vi "ATF-Storage-DI Cumulative Sequence Check.vi"(6 "output cluster":T1, 9 "CDT":dbl, 11 "Numeric 2":i32) -> (1 "Failure case Seq":string, 2 "Boolean":bool, 3 "String":string)   [LabVIEW 2022 SP3]
uses:
  RT Controls/ATF Storage-FGV Read write.ctl
panel:
  out "Numeric":i32
  out "number":dbl
  out "x >= y?":bool
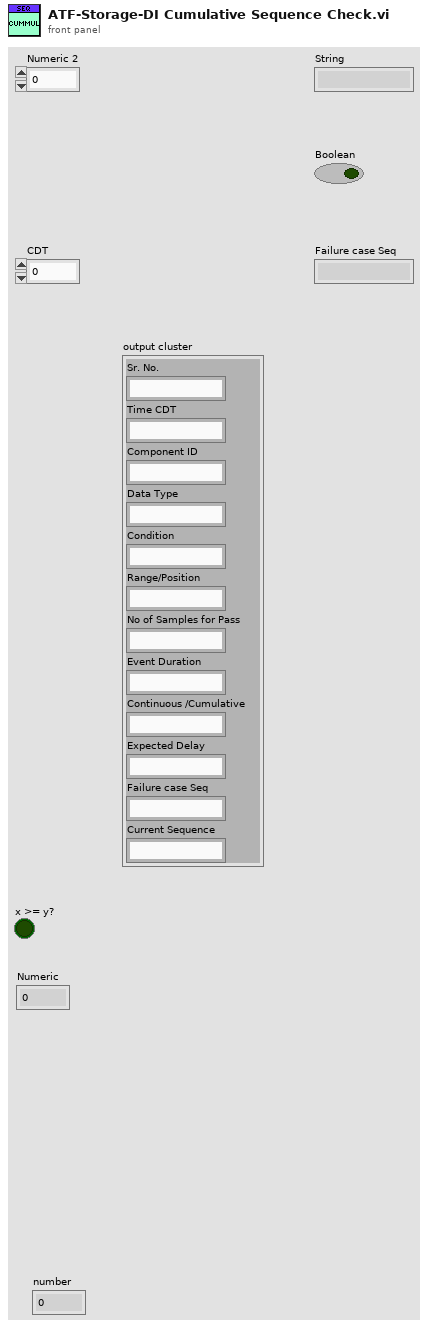
[diagram p1: front panel]
types:
  T1 = cluster{"Sr. No.":string, "Time CDT":string, "Component ID":string, "Data Type":string, "Condition":string, "Range/Position":string, "No of Samples for Pass":string, "Event Duration":string, "Continuous /Cumulative":string, "Expected Delay":string, "Failure case Seq":string, "Current Sequence":string}
  T2 = typedef "ATF Storage-FGV Read write.ctl" = enum16{"Write", "Read"}
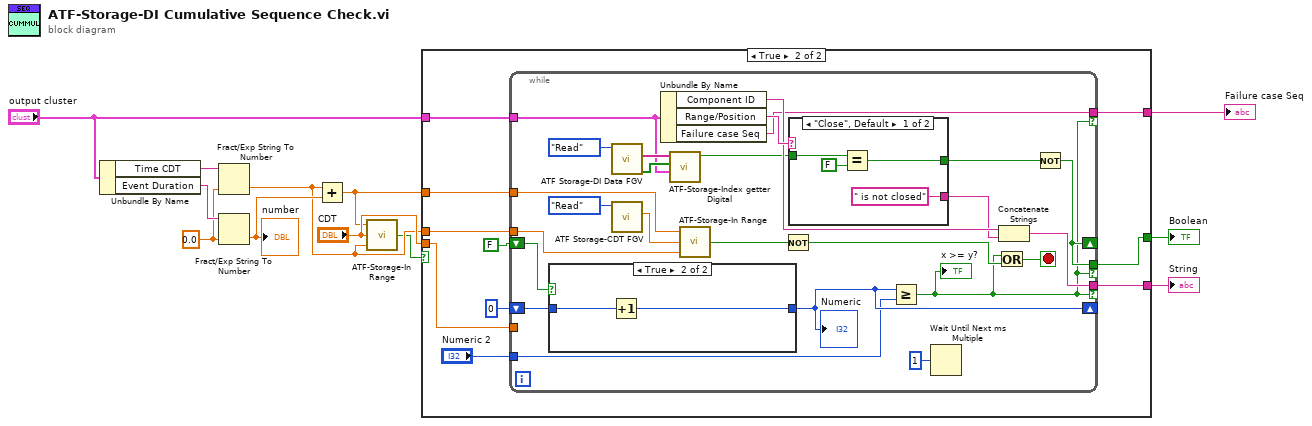
[diagram p0: block diagram]
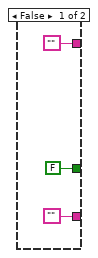
[diagram p2: hidden frame]
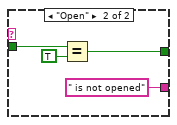
[diagram p3: hidden frame]
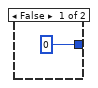
[diagram p4: hidden frame]
diagram:
  w6 = 0.0
  n1 = Unbundle By Name("output cluster") -> ("Time CDT"=w8:string, "Event Duration"=w7:string)
  n2 = Fract/Exp String To Number(string=w8, default (0 dbl)=w6) -> (number=w2:dbl)  [unwired: 2 in, 1 out]
  n3 = Fract/Exp String To Number(string=w7, default (0 dbl)=w6) -> (number=w9:dbl)  [unwired: 2 in, 1 out]
  "number" <- w9
  n4 = Add(x=w2, y=w9) -> (x+y=w3:dbl)
  n5 = call "ATF-Storage-In Range.vi"("Min"=w2, "X"="CDT", "Max"=w3) -> ("In Range"=w1:bool)  [unwired: 2 in]
  n6 = case shown="True" w1 {
    tunnel: ["" ("Empty String Constant") w25] -> w12
    tunnel: ["" ("Empty String Constant") w24] -> w11
    tunnel: [FALSE w23] -> w10
    tunnel: "output cluster" -> [_ w21]
    tunnel: "CDT" -> [_ w20]
    tunnel: w3 -> [_ w17]
    tunnel: w2 -> [_ w16]
    frame False {
    }
    frame True {
      n7 = while {
        tunnel: w21 -> [w28]
        tunnel: [w48] -> w24 if=w34
        shift-right: [w43] -> _
        shift-left: FALSE -> [w46]
        shift-right: [w45] -> _
        shift-left: 0 ("Numeric") -> [w47]
        tunnel: [w44] -> w25 if=w34
        tunnel: [w43] -> w23 if=w34
        tunnel: w20 -> [_]
        tunnel: "Numeric 2" -> [w40]
        tunnel: w17 -> [w37]
        tunnel: w16 -> [w36]
        stop <- w33 stop-if-true
        n8 = case shown="True" w46 {
          tunnel: [0 w61] -> w45
          tunnel: w47 -> [_ w60]
          frame False {
          }
          frame True {
            n9 = Increment(x=w60) -> (x+1=w61:i32)
          }
        }
        "Numeric" <- w45
        n10 = call "ATF Storage-DI Data FGV.vi"("Write/Read"=ATF_Storage-FGV_Read_write."Read") -> ("DI Y LP"=w29:bool[], "DI Signal List LP"=w30:string[])  [unwired: 8 in, 1 out]
        n11 = call "ATF Storage-CDT FGV.vi"("Write/Read"=enum16{"Write", "Read"}."Read") -> ("CDT Out"=w38:dbl)  [unwired: 9 in, 1 out]
        n12 = Unbundle By Name(w28) -> ("Component ID"=w49:string, "Range/Position"=w50:string, "Failure case Seq"=w44:string)
        n13 = call "ATF-Storage-Index getter  Digital.vi"("output cluster"=w28, "DI Y  data"=w29, "DI Channels Name"=w30) -> ("Digital data"=w27:bool)  [unwired: 8 in]
        n14 = call "ATF-Storage-In Range.vi"("Min"=w36, "X"=w38, "Max"=w37) -> ("In Range"=w32:bool)  [unwired: 2 in]
        n15 = Not(x=w32) -> (.not. x?=w35:bool)
        n16 = case shown="\"Close\", Default" w50 {
          tunnel: w27 -> [w53 w58]
          tunnel: [w51 w56] -> w42
          tunnel: [" is not closed" ("string") " is not opened" ("string")] -> w41
          frame "Close", Default {
            n17 = Equal?(x=w53, y=FALSE ("x")) -> (x = y?=w51:bool)
          }
          frame "Open" {
            n18 = Equal?(x=w58, y=TRUE ("x")) -> (x = y?=w56:bool)
          }
        }
        n19 = Greater Or Equal?(x=w45, y=w40) -> (x >= y?=w34:bool)
        "x >= y?" <- w34
        n20 = Wait Until Next ms Multiple(millisecond multiple=u32 1) -> ()  [unwired: 1 out]
        n21 = Or(x=w34, y=w35) -> (x .or. y?=w33:bool)
        n22 = Concatenate Strings(w49, w41) -> (w48:string)
        n23 = Not(x=w42) -> (.not. x?=w43:bool)
      }
    }
  }
  "Failure case Seq" <- w12
  "String" <- w11
  "Boolean" <- w10
